vi "Read Action.vi"(8 "error in (no error)":errorcluster, 11 "CONTROLLER in":refnum<class "CONTROLLER.lvclass">) -> (0 "error out":errorcluster, 2 "Action":string, 3 "CONTROLLER out":refnum<class "CONTROLLER.lvclass">)   [LabVIEW 2013, in "CONTROLLER.lvclass"]
doc: "This method will output tje action value from the class and clear its value"
uses:
  CONTROLLER.lvclass
  CONTROLLER.lvclass/CONTROLLER.ctl
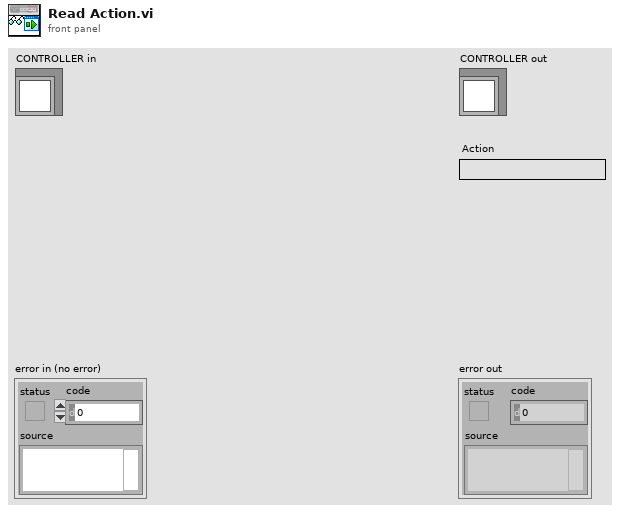
[diagram p1: front panel]
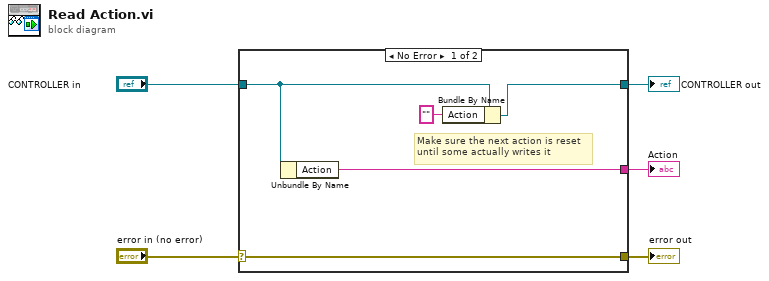
[diagram p0: block diagram]
diagram:
  n1 = case shown="No Error" "error in (no error)" {
    selector: "error in (no error)" -> [w10 w11]
    tunnel: [w10 w11] -> w4
    tunnel: [w7 w12] -> w2
    tunnel: "CONTROLLER in" -> [w8 w12]
    tunnel: [w9 _] -> w1
    frame No Error {
      # "Make sure the next action is reset\nuntil some actually writes it"
      n2 = Unbundle By Name(w8) -> ("Action"=w9:string)
      n3 = Bundle By Name(cluster=w8, "Action"="") -> (w7:refnum<class "CONTROLLER.lvclass">)
    }
    frame Error {
    }
  }
  "error out" <- w4
  "CONTROLLER out" <- w2
  "Action" <- w1
